vi "Configure Channel.vi"(8 "error in (no error)":errorcluster, 10 "DAQmx Task In":refnum<k21>, 11 "VoltageOutChannel in":refnum<class "VoltageOutChannel.lvclass">) -> (0 "error out":errorcluster, 2 "DAQmx Task":refnum<k21>)   [LabVIEW 2020, in "VolatusDAQConfig.lvlib" / "VoltageOutChannel.lvclass"]
uses:
  VoltageOutChannel.lvclass
  C:/dev/lv20CE/relink/lv-volatus/VolatusConfig/VolatusConfigElement/VolatusConfigElement.lvclass
  C:/dev/lv20CE/relink/lv-volatus/VolatusConfig/Channel/Channel.lvclass
  VolatusConfig/VolatusConfigElement/VolatusConfigElement.lvclass/VolatusConfigElement.ctl
  VolatusConfig/VolatusConfigElement/Element.vi
  VolatusConfig/VolatusConfigElement/Lookup Child by Name.vi
  VolatusConfig/Channel/Channel Config.lvclass
  lv-cdm/CDM-Config/Config Element/Lookup Child by Name.vi
  lv-cdm/CDM-Config/Config Element/Value (String).vi
  <vilib>/DAQmx/create/channels.llb/DAQmx Create Channel (AO-Voltage-Basic).vi
  VoltageOutChannel.lvclass/VoltageOutChannel.ctl
  C:/dev/lv20CE/relink/lv-volatus/VolatusDAQConfig/DAQmxChannel/DAQmxChannel.lvclass
  C:/dev/lv20CE/relink/lv-volatus/VolatusConfig/Channel/Channel Config.lvclass
  C:/dev/lv20CE/relink/lv-volatus/VolatusDAQConfig/VoltageOutChannel/VoltageOutChannel.lvclass
  VolatusConfig/VolatusConfigElement/VolatusConfigElement.lvclass
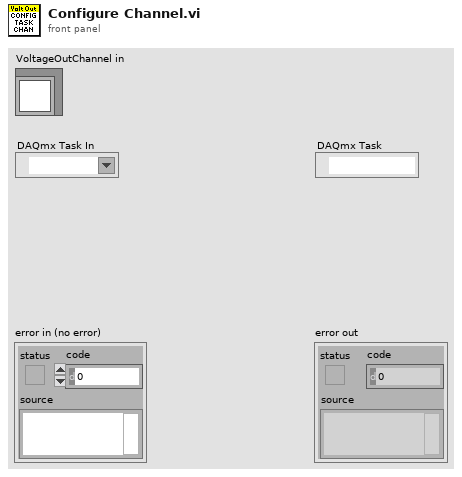
[diagram p1: front panel]
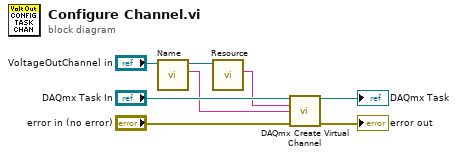
[diagram p0: block diagram]
diagram:
  n1 = call "Name.vi"("VolatusConfigElement in"="VoltageOutChannel in") -> ("Name"=w1:string, "VolatusConfigElement out"=w2:refnum<class "VoltageOutChannel.lvclass">)  [unwired: 8 in, 1 out]
  n2 = call "Resource.vi"("Channel in"=w2) -> ("Resource"=w3:string)  [unwired: 8 in, 2 out]
  n3 = call-poly <vilib>:"DAQmx Create Virtual Channel.vi"("task in"="DAQmx Task In", "physical channels"=w3, "name to assign"=w1, "error in"="error in (no error)") -> ("task out"=→"DAQmx Task":refnum<k21>, "error out"=→"error out":errorcluster)  [unwired: 10 in]
